vi "SetMultiLineColor.vi"(7 "色指定":cluster{"背景色":u32, "文字色":u32}, 8 "Error In":errorcluster caption="エラー入力", 9 "長さ(1)":i32=1, 10 "開始行(0)":i32, 11 "Tbl refnum":refnum<vi>) -> (0 "Error Out":errorcluster caption="エラー出力", 3 "Tbl refnum出力":refnum<vi>)   [LabVIEW 2016]
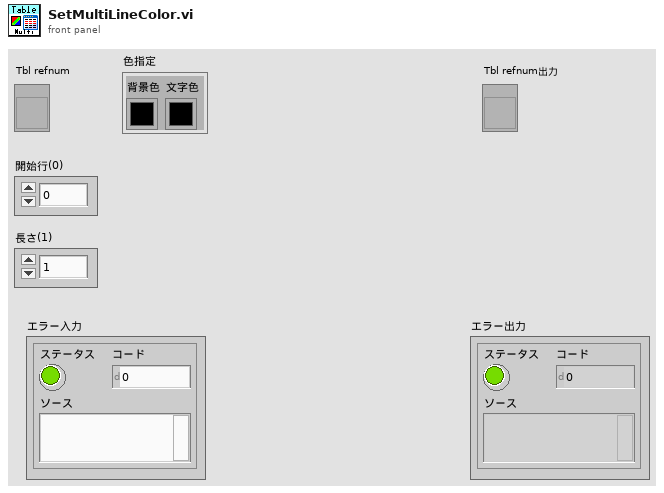
[diagram p1: front panel]
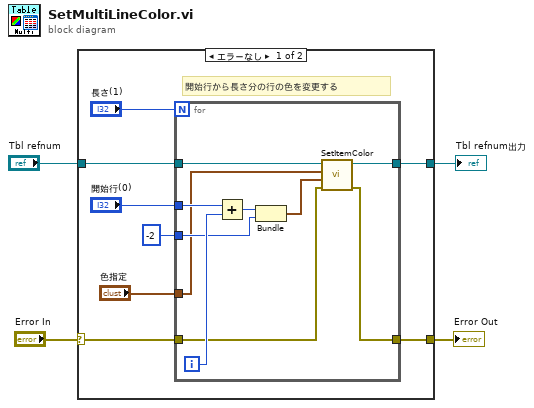
[diagram p0: block diagram]
diagram:
  n1 = case shown="エラーなし" "Error In" {
    selector: "Error In" -> [w8 w24]
    tunnel: [w7 w24] -> w3
    tunnel: "Tbl refnum" -> [w6 w23]
    tunnel: [w5 w23] -> w1
    frame No Error {
      # "開始行から長さ分の行の色を変更する"
      n2 = for {
        N: "長さ(1)" -> [_]
        tunnel: w6 -> [w14]
        tunnel: "開始行(0)" -> [w22]
        tunnel: -2 -> [w19]
        tunnel: "色指定" -> [w17]
        tunnel: w8 -> [w16]
        tunnel: [w15] -> w7
        tunnel: [w13] -> w5
        i -> [w21]
        n3 = Add(x=w22, y=w21) -> (x+y=w20:i32)
        n4 = Bundle(w20, w19) -> (w18:cluster{i32, i32})  [unwired: 1 in]
        n5 = call "SetItemColor.vi"("エラー入力(エラーなし)"=w16, "行列指定"=w18, "色指定"=w17, "Tbl refnum"=w14) -> ("エラー出力"=w15:errorcluster, "Tbl refnum出力"=w13:refnum<vi>)  [unwired: 6 in]
      }
    }
    frame Error {
    }
  }
  "Error Out" <- w3
  "Tbl refnum出力" <- w1
